vi "Auto Sequence 2.vi"   [LabVIEW 2014]
types:
  T1 = cluster{"proportional gain (Kc)":dbl, "integral time (Ti, min)":dbl, "derivative time (Td, min)":dbl}
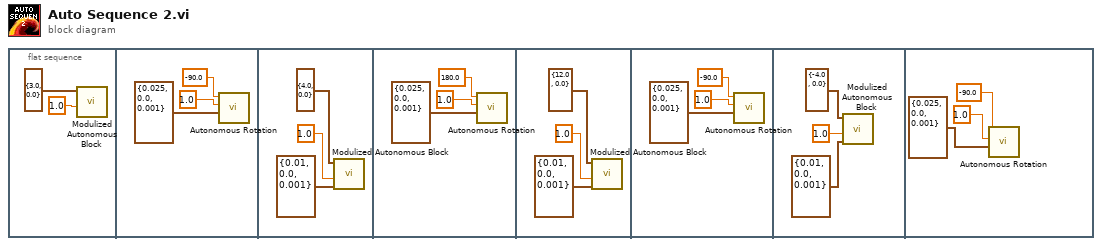
[diagram p0: block diagram]
diagram:
  n1 = flat-sequence {
    frame #0 {
      n2 = call "Modulized Autonomous Block.vi"("Power"=1.0, "auto Coords"=cluster{"X":dbl, "Y":dbl} {"X"=3.0, "Y"=0.0}) -> ()  [unwired: 9 in, 1 out]
    }
    frame #1 {
      n3 = call "Autonomous Rotation.vi"("PID gains"=T1 {"proportional gain (Kc)"=0.025, "integral time (Ti, min)"=0.0, "derivative time (Td, min)"=0.001}, "Rotation Speed"=1.0, "Desired Angle"=-90.0) -> ()  [unwired: 9 in]
    }
    frame #2 {
      n4 = call "Modulized Autonomous Block.vi"("PID gains"=T1 {"proportional gain (Kc)"=0.01, "integral time (Ti, min)"=0.0, "derivative time (Td, min)"=0.001}, "Power"=1.0, "auto Coords"=cluster{"X":dbl, "Y":dbl} {"X"=4.0, "Y"=0.0}) -> ()  [unwired: 8 in, 1 out]
    }
    frame #3 {
      n5 = call "Autonomous Rotation.vi"("PID gains"=T1 {"proportional gain (Kc)"=0.025, "integral time (Ti, min)"=0.0, "derivative time (Td, min)"=0.001}, "Rotation Speed"=1.0, "Desired Angle"=180.0) -> ()  [unwired: 9 in]
    }
    frame #4 {
      n6 = call "Modulized Autonomous Block.vi"("PID gains"=T1 {"proportional gain (Kc)"=0.01, "integral time (Ti, min)"=0.0, "derivative time (Td, min)"=0.001}, "Power"=1.0, "auto Coords"=cluster{"X":dbl, "Y":dbl} {"X"=12.0, "Y"=0.0}) -> ()  [unwired: 8 in, 1 out]
    }
    frame #5 {
      n7 = call "Autonomous Rotation.vi"("PID gains"=T1 {"proportional gain (Kc)"=0.025, "integral time (Ti, min)"=0.0, "derivative time (Td, min)"=0.001}, "Rotation Speed"=1.0, "Desired Angle"=-90.0) -> ()  [unwired: 9 in]
    }
    frame #6 {
      n8 = call "Modulized Autonomous Block.vi"("PID gains"=T1 {"proportional gain (Kc)"=0.01, "integral time (Ti, min)"=0.0, "derivative time (Td, min)"=0.001}, "Power"=1.0, "auto Coords"=cluster{"X":dbl, "Y":dbl} {"X"=-4.0, "Y"=0.0}) -> ()  [unwired: 8 in, 1 out]
    }
    frame #7 {
      n9 = call "Autonomous Rotation.vi"("PID gains"=T1 {"proportional gain (Kc)"=0.025, "integral time (Ti, min)"=0.0, "derivative time (Td, min)"=0.001}, "Rotation Speed"=1.0, "Desired Angle"=-90.0) -> ()  [unwired: 9 in]
    }
  }
